vi "FPGAController_v4.2.vi"() -> ()   [LabVIEW 2015]
uses:
  <vilib>/Utility/miscctls.llb/LVPointTypeDef.ctl
  <vilib>/FPGAPlugInAG/PXIe-7971R/niLvFpga_Open_PXIe-7971R.vi
  <userlib>/_OpenG.lib/file/file.llb/Strip Path Extension - Path__ogtk.vi
  <userlib>/_OpenG.lib/comparison/comparison.llb/DBL Changed__ogtk.vi
  <userlib>/_OpenG.lib/comparison/comparison.llb/Boolean Changed__ogtk.vi
  <vilib>/Utility/error.llb/Error Cluster From Error Code.vi
  <vilib>/rvi/errors/niLvFpgaAdjustHostInterfaceError.vi
  <vilib>/addons/database/Connection.llb/Conn Execute.vi
  <vilib>/addons/database/Recordset.llb/Rec Fetch Recordset Data (R).vi
  <vilib>/addons/database/Recordset.llb/Rec Destroy - Connection.vi
  <vilib>/FPGAPlugInAG/PXIe-7971R/niLvFpga_Close_PXIe-7971R.vi
  <vilib>/rvi/interface/nirviOpenFPGA/nirviOpenFPGA.xnode
  FPGA Bitfiles/FPGAnew_FPGATarget_FPGAcode2_56iu3K9+1SM.lvbitx
  <vilib>/rvi/interface/nirviMethod/nirviMethod.xnode
  <vilib>/FPGA/interface/niFpgaViExecutionMode.ctl
  <vilib>/rvi/interface/nirviReadWriteControl/nirviReadWriteControl.xnode
  <vilib>/addons/database/_DB Variant To Data/Database Variant To Data.xnode
  <vilib>/rvi/interface/nirviCloseFPGA/nirviCloseFPGA.xnode
  <vilib>/addons/database/NI_Database_API.lvlib
  NiFpgaLv.dll
panel:
  in  "Tab Control":enum32{"Auto Threshold", "Manual Threshold"}(tab)
  in  "Refresh PSU":bool=TRUE
  in  "Auto Threshold":bool
  in  "Update All":bool
  in  "Raise Threshold":bool
  in  "Lower Threshold":bool
  in  "Threshold 1":bool
  in  "Threshold 2":bool
  in  "Threshold 3":bool
  in  "Threshold 4":bool
  in  "Threshold 5":bool
  in  "Threshold 6":bool
  in  "Threshold 7":bool
  in  "Update By":i32
  out "Time Betwee Shots":dbl
  out "Del Armed":bool
  out "Update Threshold":bool
  in  "Min. Time\nBetween Shots (s)":dbl
  in  "Rate Limiting":bool
  out "Armed":bool
  in  "Add Delay":bool
  in  "Delay Name":string
  in  "Delay Value":dbl=3.0 min=0.0
  in  "Delay Ring":dbl(ring)=3.15039 items=["Custom"]
  in  "Rearm Trigger":bool
  in  "One Shot Mode":bool
  out "Last Update:":timestamp
  out "Updating FPGA":bool
  out "Sensitivity":dbl
  out "error out":errorcluster
  out "Low Mass Limit":fxp<+,31,17>
  out "High Mass Limit":fxp<+,31,17>
  out "stopping":bool
  out "Peletron (MV)":dbl=2.0
  out "High Mass (kg)":dbl=inf
  out "Low Mass (kg)":dbl
  out "High Charge Limit":i16
  out "Low Charge Limit":i16
  out "High velocity count":i32=210
  out "Low velocity count":i32=21000
  in  "stop":bool
  in  "Peak-Threshold Factor":dbl=2.0
  out "Low Charge Limit (fC)":dbl
  out "High Charge Limit (fC)":dbl=100.0
  out "High Velocity":dbl=100000.0
  out "Low Velocity":dbl=1000.0
  out "Filter 7 Peak":i32=7483
  out "Filter 6 Peak":i32=9863
  out "Filter 5 Peak":i32=13910
  out "Filter 4 Peak":i32=18191
  out "Filter 3 Peak":i32=46254
  out "Filter 2 Peak":i32=120664
  out "Filter 1 Peak":i32=295996
  in  "Filter7 Threshold":i32=-21165
  in  "Filter6 Threshold":i32=-29358
  in  "Filter5 Threshold":i32=-41730
  in  "Filter4 Threshold":i32=-54306
  in  "Filter3 Threshold":i32=-138762
  in  "Filter2 Threshold":i32=-361992
  in  "Filter1 Threshold":i32=-887988
  in  "Zero Peak Values":bool
  in  "Assign Threshold":bool
  in  "Run Mode":bool
  # "Settings"
  # "Dubugging"
  # "Independent Variable"
  # "Low Vel."
  # "High Vel."
  # "Low Q (fC)"
  # "High Q (fC)"
  # "Plate Control While Loop Counter"
  # "Low Mass (kg)"
  # "High Mass (kg)"
  # "Sens. (V/pC)"
  # "Peletron (MV)"
  # "Current Value of Running Average"
  # "Peak Threshold Factor"
  # "Delay Trigger"
  # "Dist. from 2nd Det. (m)"
  # "Name"
  # "Peak Values"
  # "Peak 1"
  # "Peak 2"
  # "Peak 3"
  # "Peak 4"
  # "Peak 5"
  # "Peak 6"
  # "Peak 7"
  # "Thresholds"
  # "Threshold 1"
  # "Threshold 2"
  # "Threshold 3"
  # "Threshold 4"
  # "Threshold 5"
  # "Threshold 6"
  # "Threshold 7"
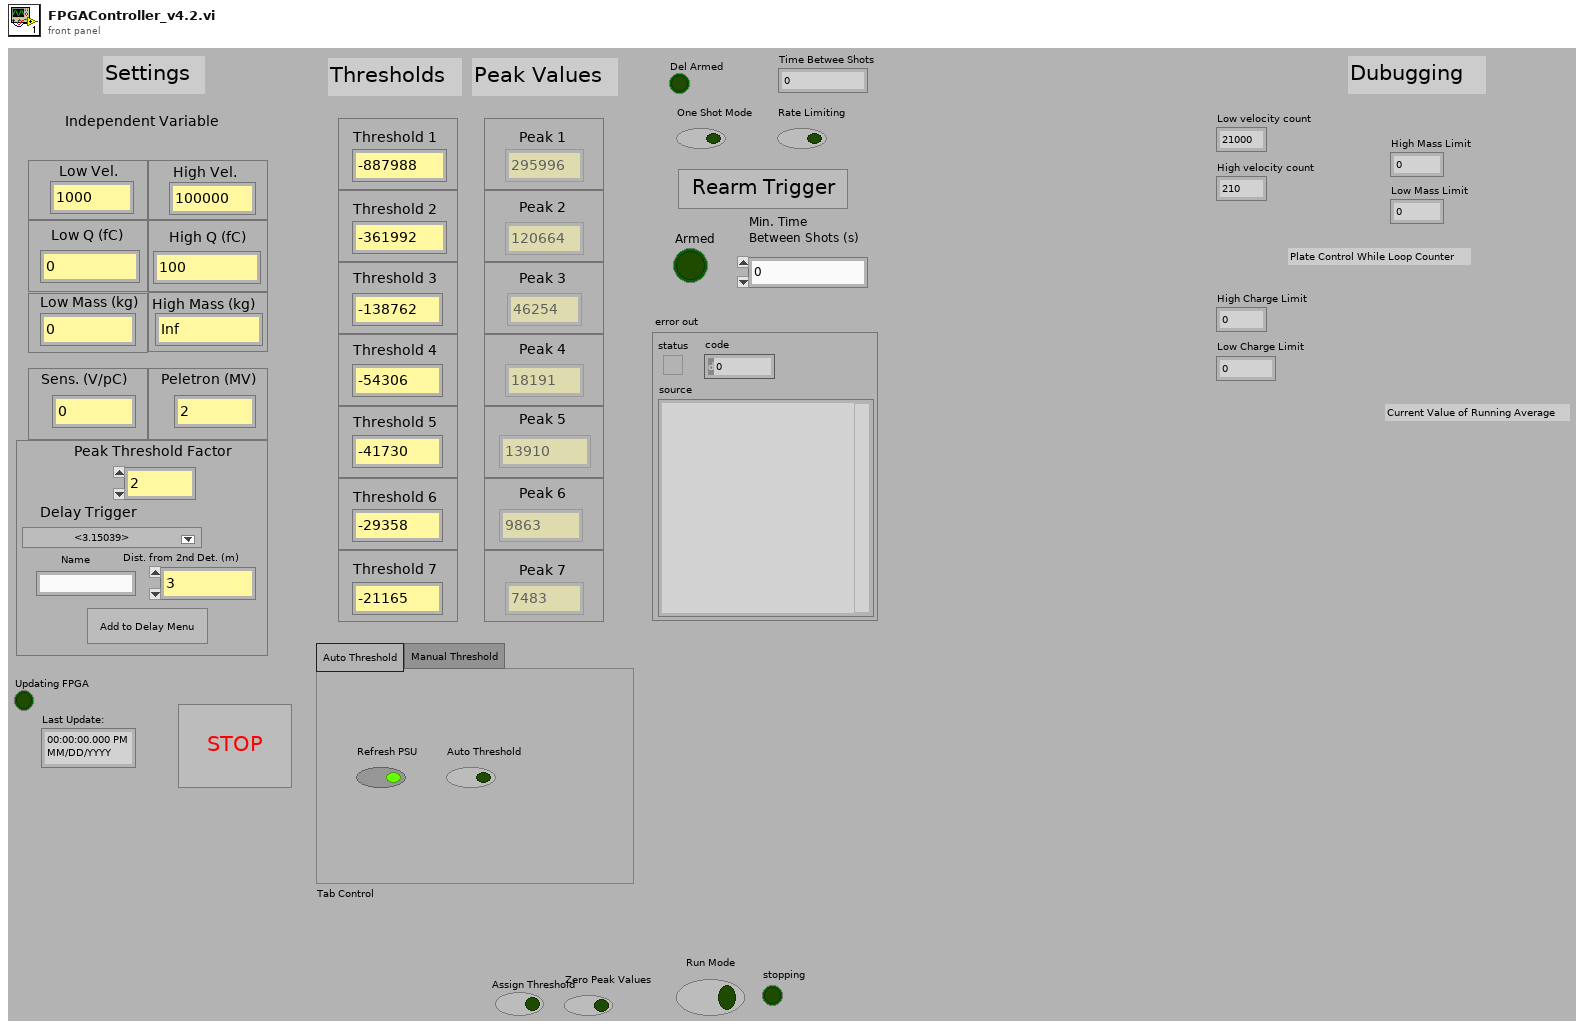
[diagram p1: front panel]
types:
  T1 = typedef "LVPointTypeDef.ctl" = cluster{"Horizontal":i16, "Vertical":i16}
  T2 = enum8{"Enabled", "Disabled", "Disabled and Grayed Out"}
  T3 = typedef "NI_Database_API.lvlib/Conn ObjectReference.ctl" = refnum<k1>
  T4 = typedef "NI_Database_API.lvlib/Rec ObjectReference.ctl" = refnum<k1>
  T5 = cluster{"Filter 1 Peak":i32, "Filter 2 Peak":i32, "Filter 3 Peak":i32, "Filter 4 Peak":i32, "Filter 5 Peak":i32, "Filter 6 Peak":i32, "Filter 7 Peak":i32}
  T6 = typedef "LVStringsAndValuesArrayTypeDef_DBL.ctl" = cluster{"String":string, "Value":dbl}[]
  T7 = cluster{"Numeric":dbl, "Numeric":dbl, "Numeric":dbl, "Numeric":dbl, "Numeric":dbl, "Numeric":dbl, i32, dbl, "Value":dbl, fxp<+,16,7>, bool}
  T8 = cluster{"Low Velocity Count":i32, "High Velocity Count":i32, "Low Charge Limit (ADC ticks)":i16, "High Charge Limit (ADC ticks)":i16, "Low Mass (ADC*cycle^2)":i64, "High Mass (ADC*cycle^2)":i64, "Mult":fxp<+,16,7>, "Mult Use?":bool}
  T9 = cluster{"Filter 1 Detector 3 Correlation":i32, "Filter 2 Detector 3 Correlation":i32, "Filter 3 Detector 3 Correlation":i32, "Filter 4 Detector 3 Correlation":i32, "Filter 5 Detector 3 Correlation":i32, "Filter 6 Detector 3 Correlation":i32, "Filter 7 Detector 3 Correlation":i32}
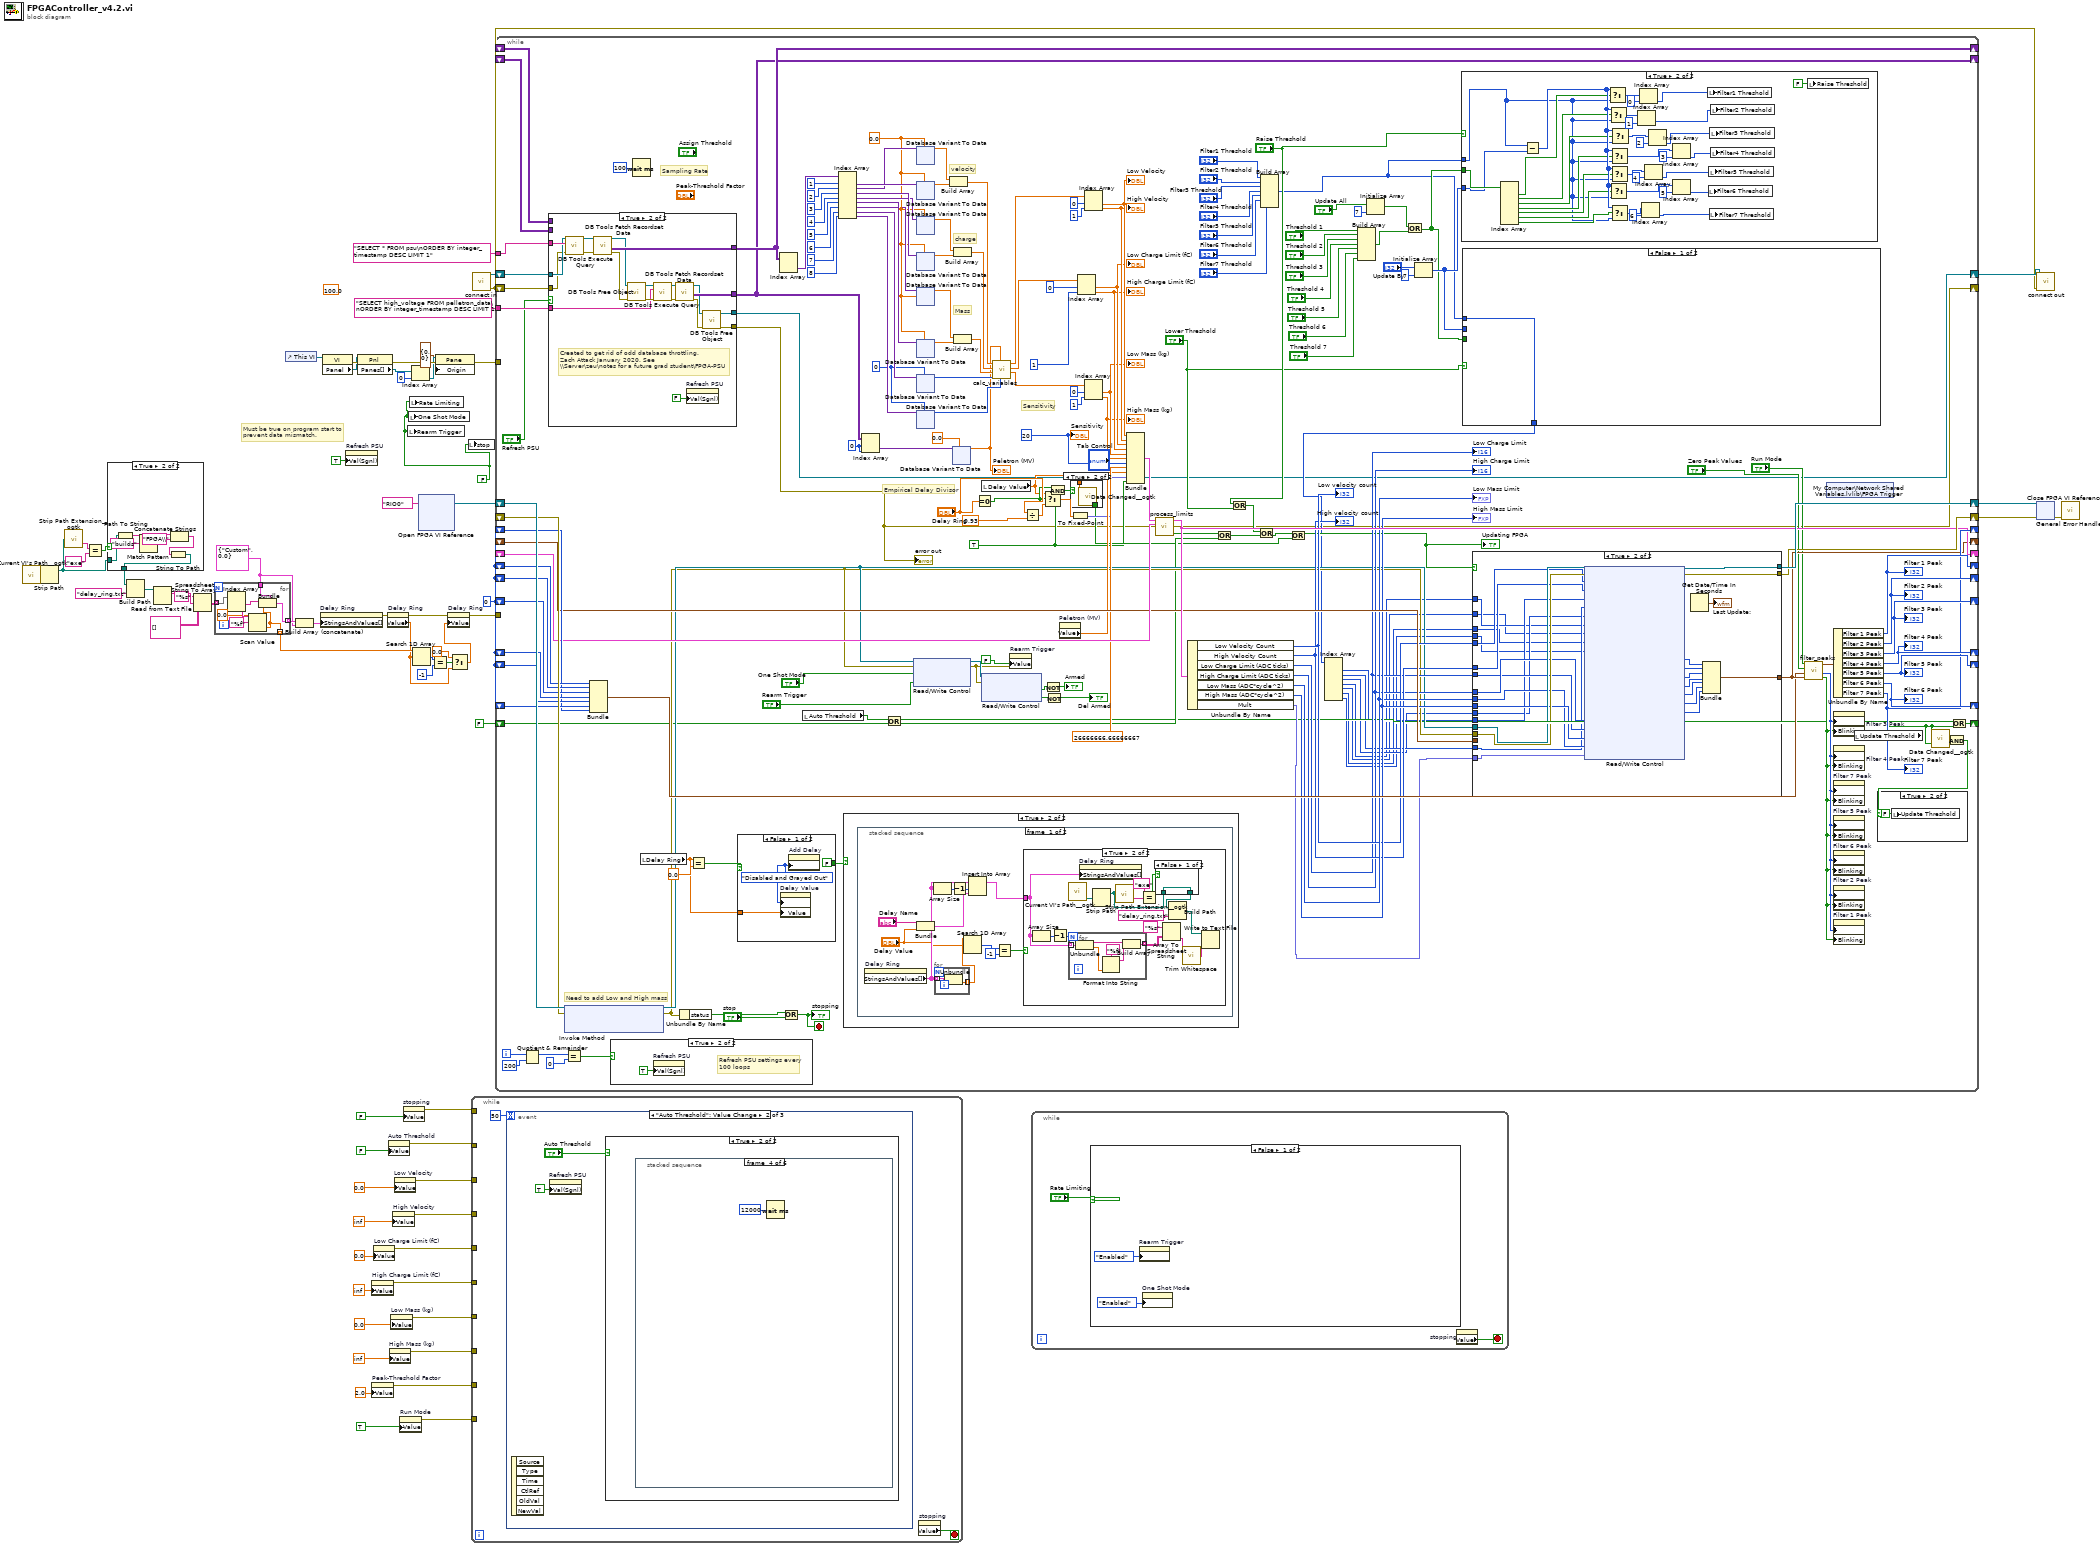
[diagram p0: block diagram]
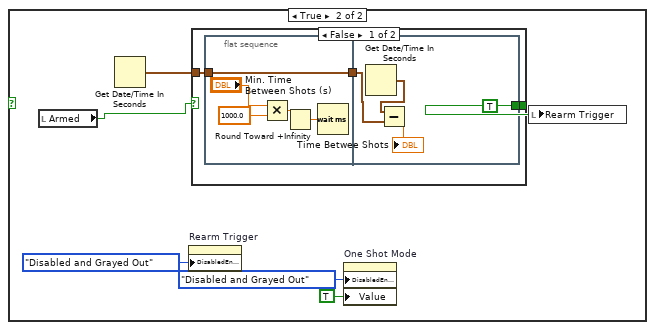
[diagram p3: hidden frame]
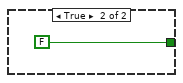
[diagram p4: hidden frame]
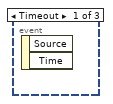
[diagram p5: hidden frame]
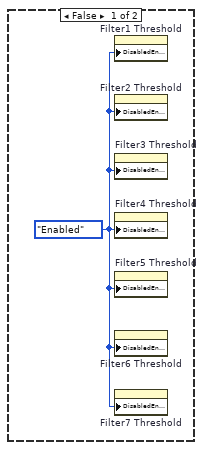
[diagram p6: hidden frame]
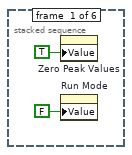
[diagram p7: hidden frame]
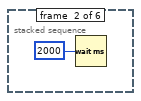
[diagram p8: hidden frame]
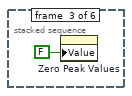
[diagram p9: hidden frame]
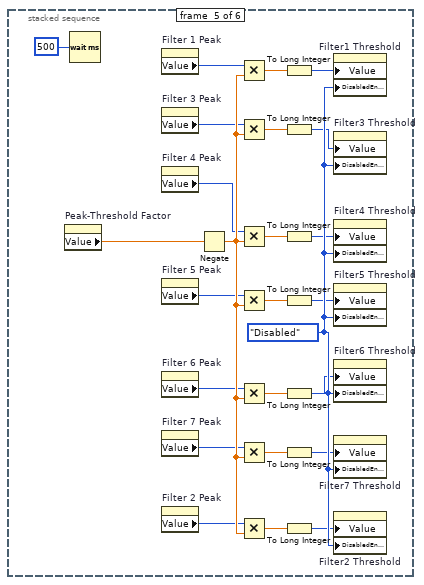
[diagram p10: hidden frame]
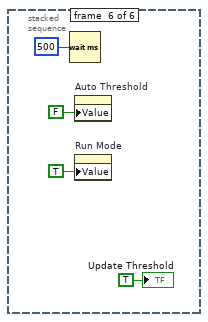
[diagram p11: hidden frame]
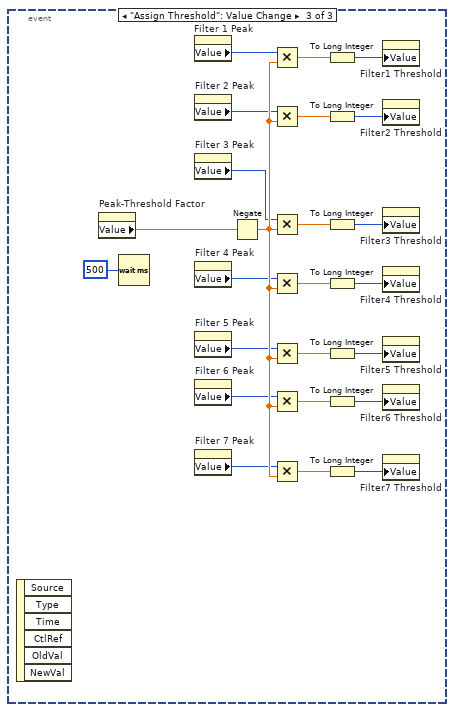
[diagram p12: hidden frame]
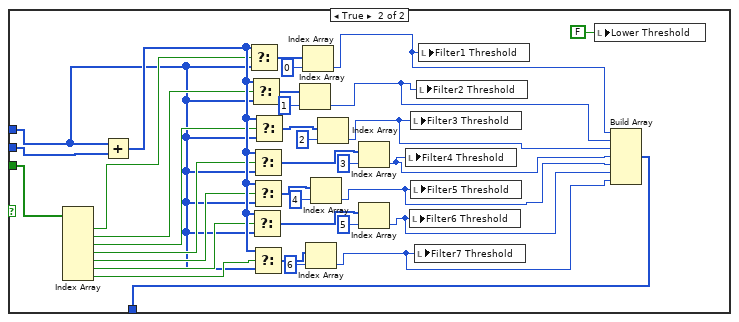
[diagram p15: hidden frame]
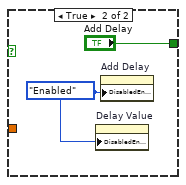
[diagram p19: hidden frame]
diagram:
  (unwired) 100.0 ("Update By")
  w19 = cluster{"String":string, "Value":dbl} {"String"="Custom", "Value"=0.0}
  w29 = FALSE
  w67 = 0
  # "Must be true on program start to\nprevent data mismatch."
  n1 = call <userlib>:"Current VI's Path__ogtk.vi"() -> ("Current VI's Path (+ Relative)"=w28:path)  [unwired: 1 in]
  n2 = Strip Path(path=w28) -> (stripped path=w14:path)  [unwired: 1 out]
  n3 = call-poly <userlib>:"Strip Path Extension__ogtk.vi"("path"=w14) -> ("extension"=w18:string)  [unwired: 1 out]
  n4 = Equal?(x=w18, y="exe") -> (x = y?=w15:bool)
  n5 = case shown="True" w15 {
    tunnel: w14 -> [w69 w76]
    tunnel: [w69 w70] -> w13
    frame False {
    }
    frame True {
      n6 = Path To String(path=w76) -> (string=w75:string)
      n7 = Match Pattern(string=w75, regular expression="builds") -> (before substring=w73:string)  [unwired: 1 in, 3 out]
      n8 = Concatenate Strings(w73, "FPGA\\" ("string")) -> (w71:string)
      n9 = String To Path(string=w71) -> (path=w70:path)
    }
  }
  n10 = Build Path(base path=w13, name or relative path="delay_ring.txt") -> (appended path=w16:path)
  n11 = Read from Text File(file (use dialog)=w16) -> (text=w26:string)  [unwired: 3 in, 3 out]
  n12 = Spreadsheet String To Array(format string="%s", spreadsheet string=w26, array type (2D Dbl)=string[][] []) -> (array=w23:string[][])  [unwired: 1 in]
  n13 = for {
    tunnel: w23 -> [w84] mode=indexing
    tunnel: w19 -> [w82]
    tunnel: [w78] -> w20 mode=indexing
    tunnel: [w77] -> w12 mode=indexing
    n14 = Index Array(array=w84) -> (element #1=w83:string, element #2=w81:string)  [unwired: 2 in]
    n15 = Scan Value(string=w81, format string="%f", default (0 dbl)=0.0) -> (value=w77:dbl)  [unwired: 1 out]
    n16 = Bundle(cluster=w82, "String"=w83, "Value"=w77) -> (w78:cluster{"String":string, "Value":dbl})
  }
  n17 = control-ref of="This VI"() -> (w40:refnum<vi>)
  n18 = Build Array (concatenate)(w20, w19) -> (w22:cluster{"String":string, "Value":dbl}[])
  n19 = property on="Delay Ring" class="Ring (strict)"("StringsAndValues[]"=w22) -> (error out=w21:errorcluster)  [unwired: 2 in, 1 out]
  n20 = property class="VI"(reference=w40) -> (error out=w39:errorcluster, "Panel"=w38:refnum<vi>)  [unwired: 1 in, 1 out]
  n21 = property on="Refresh PSU" class="Bool (strict)"("Val(Sgnl)"=TRUE ("Value (Signaling)")) -> ()  [unwired: 2 in, 2 out]
  n22 = property class="Pnl"(reference=w38, error in=w39) -> (error out=w37:errorcluster, "Panes[]"=w36:refnum<vi>[])  [unwired: 1 out]
  n23 = property on="High Charge Limit (fC)" class="DigNum (strict)"("Value"=inf ("High Charge Limit (fC)")) -> (error out=w54:errorcluster)  [unwired: 2 in, 1 out]
  n24 = property on="Peak-Threshold Factor" class="DigNum (strict)"("Value"=2.0 ("Peak-Threshold Factor")) -> (error out=w48:errorcluster)  [unwired: 2 in, 1 out]
  n25 = property on="Low Charge Limit (fC)" class="DigNum (strict)"("Value"=0.0 ("Low Charge Limit (fC)")) -> (error out=w56:errorcluster)  [unwired: 2 in, 1 out]
  n26 = property on="Delay Ring" class="Ring (strict)"(error in=w21) -> (error out=w11:errorcluster, "Value"=w5:dbl)  [unwired: 1 in, 1 out]
  n27 = property on="Auto Threshold" class="Bool (strict)"("Value"=FALSE ("Auto Threshold")) -> (error out=w62:errorcluster)  [unwired: 2 in, 1 out]
  n28 = property on="High Mass (kg)" class="DigNum (strict)"("Value"=inf ("High Mass (kg)")) -> (error out=w50:errorcluster)  [unwired: 2 in, 1 out]
  n29 = property on="Low Mass (kg)" class="DigNum (strict)"("Value"=0.0 ("Low Mass (kg)")) -> (error out=w52:errorcluster)  [unwired: 2 in, 1 out]
  n30 = property on="High Velocity" class="DigNum (strict)"("Value"=inf ("High Velocity")) -> (error out=w58:errorcluster)  [unwired: 2 in, 1 out]
  n31 = property on="Low Velocity" class="DigNum (strict)"("Value"=0.0 ("Low Velocity")) -> (error out=w60:errorcluster)  [unwired: 2 in, 1 out]
  n32 = property on="Run Mode" class="Bool (strict)"("Value"=TRUE ("Run Mode")) -> (error out=w46:errorcluster)  [unwired: 2 in, 1 out]
  n33 = property on="stopping" class="Bool (strict)"("Value"=FALSE ("stopping")) -> (error out=w64:errorcluster)  [unwired: 2 in, 1 out]
  n34 = local write "Rearm Trigger"(w29) -> ()
  n35 = local write "One Shot Mode"(w29) -> ()
  n36 = local write "Rate Limiting"(w29) -> ()
  n37 = Index Array(array=w36, index=0) -> (element=w34:refnum<vi>)
  n38 = Search 1D Array(1D array=w12, element=w5) -> (index of element=w9:i32)  [unwired: 1 in]
  n39 = xnode "Open FPGA VI Reference"("resource name"=tag "RIO0") -> ("FPGA VI Reference Out"=w31:refnum<k20>)  [unwired: 1 in, 1 out]
  n40 = Equal?(x=w9, y=-1) -> (x = y?=w7:bool)
  n41 = property class="Pane"(reference=w34, error in=w37, "Origin"=T1 {"Horizontal"=0, "Vertical"=0}) -> (error out=w32:errorcluster)  [unwired: 1 out]
  n42 = Select(t=0.0, s=w7, f=w5) -> (s? t:f=w6:dbl)
  n43 = property on="Delay Ring" class="Ring (strict)"(error in=w11, "Value"=w6) -> (error out=w10:errorcluster)  [unwired: 1 in, 1 out]
  n44 = local write "stop"(w29) -> ()
  n45 = while {
    tunnel: w64 -> [_]
    tunnel: w62 -> [_]
    tunnel: w60 -> [_]
    tunnel: w58 -> [_]
    tunnel: w56 -> [_]
    tunnel: w54 -> [_]
    tunnel: w52 -> [_]
    tunnel: w50 -> [_]
    tunnel: w48 -> [_]
    tunnel: w46 -> [_]
    stop <- w86 stop-if-true
    n46 = event shown="[1] \"Auto Threshold\": Value Change" {
      selector: _ -> [_ _ _]
      dyn-events: _ -> [_ _ _]
      timeout: 50 -> [_ _ _]
      event Timeout {
        n47 = event-data() -> ()  [unwired: 1 in, 2 out]
      }
      event "Auto Threshold": Value Change {
        n48 = event-data() -> ()  [unwired: 1 in, 6 out]
        n49 = property on="Refresh PSU" class="Bool (strict)"("Val(Sgnl)"=TRUE ("Value (Signaling)")) -> ()  [unwired: 2 in, 2 out]
        n50 = case shown="True" "Auto Threshold" {
          frame False {
            w89 = T2."Enabled" ("Disabled")
            n51 = property on="Filter1 Threshold" class="DigNum (strict)"("DisabledEnum"=w89) -> ()  [unwired: 2 in, 2 out]
            n52 = property on="Filter2 Threshold" class="DigNum (strict)"("DisabledEnum"=w89) -> ()  [unwired: 2 in, 2 out]
            n53 = property on="Filter3 Threshold" class="DigNum (strict)"("DisabledEnum"=w89) -> ()  [unwired: 2 in, 2 out]
            n54 = property on="Filter4 Threshold" class="DigNum (strict)"("DisabledEnum"=w89) -> ()  [unwired: 2 in, 2 out]
            n55 = property on="Filter5 Threshold" class="DigNum (strict)"("DisabledEnum"=w89) -> ()  [unwired: 2 in, 2 out]
            n56 = property on="Filter6 Threshold" class="DigNum (strict)"("DisabledEnum"=w89) -> ()  [unwired: 2 in, 2 out]
            n57 = property on="Filter7 Threshold" class="DigNum (strict)"("DisabledEnum"=w89) -> ()  [unwired: 2 in, 2 out]
          }
          frame True {
            n58 = stacked-sequence {
              frame #0 {
                n59 = property on="Zero Peak Values" class="Bool (strict)"("Value"=TRUE ("Zero Peak Values")) -> ()  [unwired: 2 in, 2 out]
                n60 = property on="Run Mode" class="Bool (strict)"("Value"=FALSE ("Run Mode")) -> ()  [unwired: 2 in, 2 out]
              }
              frame #1 {
                n61 = Wait (ms)(milliseconds to wait=u32 2000) -> ()  [unwired: 1 out]
              }
              frame #2 {
                n62 = property on="Zero Peak Values" class="Bool (strict)"("Value"=FALSE ("Zero Peak Values")) -> ()  [unwired: 2 in, 2 out]
              }
              frame #3 {
                n63 = Wait (ms)(milliseconds to wait=u32 12000) -> ()  [unwired: 1 out]
              }
              frame #4 {
                w119 = T2."Disabled" ("Disabled")
                n64 = property on="Peak-Threshold Factor" class="DigNum (strict)"() -> ("Value"=w104:dbl)  [unwired: 2 in, 2 out]
                n65 = Wait (ms)(milliseconds to wait=u32 500) -> ()  [unwired: 1 out]
                n66 = property on="Filter 1 Peak" class="DigNum (strict)"() -> ("Value"=w102:i32)  [unwired: 2 in, 2 out]
                n67 = property on="Filter 3 Peak" class="DigNum (strict)"() -> ("Value"=w100:i32)  [unwired: 2 in, 2 out]
                n68 = property on="Filter 4 Peak" class="DigNum (strict)"() -> ("Value"=w99:i32)  [unwired: 2 in, 2 out]
                n69 = property on="Filter 5 Peak" class="DigNum (strict)"() -> ("Value"=w98:i32)  [unwired: 2 in, 2 out]
                n70 = property on="Filter 6 Peak" class="DigNum (strict)"() -> ("Value"=w97:i32)  [unwired: 2 in, 2 out]
                n71 = property on="Filter 7 Peak" class="DigNum (strict)"() -> ("Value"=w96:i32)  [unwired: 2 in, 2 out]
                n72 = property on="Filter 2 Peak" class="DigNum (strict)"() -> ("Value"=w101:i32)  [unwired: 2 in, 2 out]
                n73 = Negate(x=w104) -> (-x=w103:dbl)
                n74 = Multiply(x=w102, y=w103) -> (x*y=w118:dbl)
                n75 = Multiply(x=w100, y=w103) -> (x*y=w114:dbl)
                n76 = Multiply(x=w99, y=w103) -> (x*y=w112:dbl)
                n77 = Multiply(x=w98, y=w103) -> (x*y=w110:dbl)
                n78 = Multiply(x=w97, y=w103) -> (x*y=w108:dbl)
                n79 = Multiply(x=w96, y=w103) -> (x*y=w106:dbl)
                n80 = Multiply(x=w101, y=w103) -> (x*y=w116:dbl)
                n81 = To Long Integer(number=w118) -> (32bit integer=w117:i32)
                n82 = To Long Integer(number=w114) -> (32bit integer=w113:i32)
                n83 = To Long Integer(number=w112) -> (32bit integer=w111:i32)
                n84 = To Long Integer(number=w110) -> (32bit integer=w109:i32)
                n85 = To Long Integer(number=w108) -> (32bit integer=w107:i32)
                n86 = To Long Integer(number=w106) -> (32bit integer=w105:i32)
                n87 = To Long Integer(number=w116) -> (32bit integer=w115:i32)
                n88 = property on="Filter1 Threshold" class="DigNum (strict)"("Value"=w117, "DisabledEnum"=w119) -> ()  [unwired: 2 in, 2 out]
                n89 = property on="Filter3 Threshold" class="DigNum (strict)"("Value"=w113, "DisabledEnum"=w119) -> ()  [unwired: 2 in, 2 out]
                n90 = property on="Filter4 Threshold" class="DigNum (strict)"("Value"=w111, "DisabledEnum"=w119) -> ()  [unwired: 2 in, 2 out]
                n91 = property on="Filter5 Threshold" class="DigNum (strict)"("Value"=w109, "DisabledEnum"=w119) -> ()  [unwired: 2 in, 2 out]
                n92 = property on="Filter6 Threshold" class="DigNum (strict)"("Value"=w107, "DisabledEnum"=w119) -> ()  [unwired: 2 in, 2 out]
                n93 = property on="Filter7 Threshold" class="DigNum (strict)"("Value"=w105, "DisabledEnum"=w119) -> ()  [unwired: 2 in, 2 out]
                n94 = property on="Filter2 Threshold" class="DigNum (strict)"("Value"=w115, "DisabledEnum"=w119) -> ()  [unwired: 2 in, 2 out]
              }
              frame #5 {
                n95 = Wait (ms)(milliseconds to wait=u32 500) -> ()  [unwired: 1 out]
                n96 = property on="Auto Threshold" class="Bool (strict)"("Value"=FALSE ("Auto Threshold")) -> ()  [unwired: 2 in, 2 out]
                n97 = property on="Run Mode" class="Bool (strict)"("Value"=TRUE ("Run Mode")) -> ()  [unwired: 2 in, 2 out]
                "Update Threshold" <- TRUE ("Update Threshold")
              }
            }
          }
        }
      }
      event "Assign Threshold": Value Change {
        n98 = event-data() -> ()  [unwired: 1 in, 6 out]
        n99 = property on="Peak-Threshold Factor" class="DigNum (strict)"() -> ("Value"=w138:dbl)  [unwired: 2 in, 2 out]
        n100 = Wait (ms)(milliseconds to wait=u32 500) -> ()  [unwired: 1 out]
        n101 = property on="Filter 1 Peak" class="DigNum (strict)"() -> ("Value"=w137:i32)  [unwired: 2 in, 2 out]
        n102 = property on="Filter 2 Peak" class="DigNum (strict)"() -> ("Value"=w136:i32)  [unwired: 2 in, 2 out]
        n103 = property on="Filter 3 Peak" class="DigNum (strict)"() -> ("Value"=w135:i32)  [unwired: 2 in, 2 out]
        n104 = property on="Filter 4 Peak" class="DigNum (strict)"() -> ("Value"=w134:i32)  [unwired: 2 in, 2 out]
        n105 = property on="Filter 5 Peak" class="DigNum (strict)"() -> ("Value"=w133:i32)  [unwired: 2 in, 2 out]
        n106 = property on="Filter 6 Peak" class="DigNum (strict)"() -> ("Value"=w132:i32)  [unwired: 2 in, 2 out]
        n107 = property on="Filter 7 Peak" class="DigNum (strict)"() -> ("Value"=w131:i32)  [unwired: 2 in, 2 out]
        n108 = Negate(x=w138) -> (-x=w140:dbl)
        n109 = Multiply(x=w137, y=w140) -> (x*y=w147:dbl)
        n110 = Multiply(x=w136, y=w140) -> (x*y=w145:dbl)
        n111 = Multiply(x=w135, y=w140) -> (x*y=w144:dbl)
        n112 = Multiply(x=w134, y=w140) -> (x*y=w143:dbl)
        n113 = Multiply(x=w133, y=w140) -> (x*y=w142:dbl)
        n114 = Multiply(x=w132, y=w140) -> (x*y=w141:dbl)
        n115 = Multiply(x=w131, y=w140) -> (x*y=w146:dbl)
        n116 = To Long Integer(number=w147) -> (32bit integer=w130:i32)
        n117 = To Long Integer(number=w145) -> (32bit integer=w129:i32)
        n118 = To Long Integer(number=w144) -> (32bit integer=w128:i32)
        n119 = To Long Integer(number=w143) -> (32bit integer=w127:i32)
        n120 = To Long Integer(number=w142) -> (32bit integer=w126:i32)
        n121 = To Long Integer(number=w141) -> (32bit integer=w125:i32)
        n122 = To Long Integer(number=w146) -> (32bit integer=w124:i32)
        n123 = property on="Filter1 Threshold" class="DigNum (strict)"("Value"=w130) -> ()  [unwired: 2 in, 2 out]
        n124 = property on="Filter2 Threshold" class="DigNum (strict)"("Value"=w129) -> ()  [unwired: 2 in, 2 out]
        n125 = property on="Filter3 Threshold" class="DigNum (strict)"("Value"=w128) -> ()  [unwired: 2 in, 2 out]
        n126 = property on="Filter4 Threshold" class="DigNum (strict)"("Value"=w127) -> ()  [unwired: 2 in, 2 out]
        n127 = property on="Filter5 Threshold" class="DigNum (strict)"("Value"=w126) -> ()  [unwired: 2 in, 2 out]
        n128 = property on="Filter6 Threshold" class="DigNum (strict)"("Value"=w125) -> ()  [unwired: 2 in, 2 out]
        n129 = property on="Filter7 Threshold" class="DigNum (strict)"("Value"=w124) -> ()  [unwired: 2 in, 2 out]
      }
    }
    n130 = property on="stopping" class="Bool (strict)"() -> ("Value"=w86:bool)  [unwired: 2 in, 2 out]
  }
  n131 = call "connect in.vi"() -> ("error out"=w41:errorcluster, "Database Connection"=w42:T3)  [unwired: 7 in, 1 out]
  n132 = while {
    shift-right: [w321] -> w66
    shift-left: w31 -> [w325]
    shift-right: [w320] -> w65
    shift-left: _ -> [w324]
    shift-right: [w316] -> _
    shift-left: w67 -> [w309]
    shift-right: [w315] -> _
    shift-left: w67 -> [w308]
    shift-right: [w314] -> _
    shift-left: w67 -> [w307]
    shift-right: [w313] -> _
    shift-left: w67 -> [w306]
    shift-right: [w312] -> _
    shift-left: w67 -> [w305]
    shift-right: [w318] -> _
    shift-left: w67 -> [w311]
    shift-right: [w317] -> _
    shift-left: w67 -> [w310]
    tunnel: "SELECT * FROM psu\nORDER BY integer_timestamp DESC LIMIT 1" ("SQL query") -> [w163]
    shift-right: [w159] -> w43
    shift-left: w42 -> [w162]
    shift-right: [w158] -> _
    shift-left: w41 -> [w161]
    shift-right: [w304] -> _
    shift-left: _ -> [w303]
    shift-right: [w301] -> _
    shift-left: _ -> [w302]
    tunnel: w32 -> [_]
    tunnel: w10 -> [_]
    shift-right: [w217] -> _
    shift-left: FALSE -> [w220]
    tunnel: "SELECT high_voltage FROM pelletron_data\nORDER BY integer_timestamp DESC LIMIT 1" ("SQL query") -> [w160]
    shift-right: [w157] -> _
    shift-left: _ -> [w156]
    shift-right: [w155] -> _
    shift-left: _ -> [w154]
    i -> [w152]
    stop <- w319 stop-if-true
    w185 = TRUE
    w267 = 0 ("index (row)")
    w268 = i8 0
    w269 = 0.0
    w243 = 20
    # "charge"
    # "Empirical Delay Divisor"
    # "Mass"
    # "velocity"
    # "Sensitivity"
    # "Sampling Rate"
    # "Need to add Low and High mass"
    n133 = Quotient & Remainder(x=w152, y=200) -> (x-y*floor(x/y)=w150:i32)  [unwired: 1 out]
    n134 = case shown="True" "Refresh PSU" {
      tunnel: [w328 w347] -> w157
      tunnel: w163 -> [_ w346]
      tunnel: w162 -> [w330 w345]
      tunnel: w161 -> [w329 w344]
      tunnel: w160 -> [_ w337]
      tunnel: [w327 w336] -> w155
      tunnel: [w330 w333] -> w159
      tunnel: [w329 w332] -> w158
      tunnel: w156 -> [w328 _]
      tunnel: w154 -> [w327 _]
      frame False {
      }
      frame True {
        # "Created to get rid of odd database throttling.\nZach Attack January 2020. See \n\\\\Server\\zeu\\notes for a future grad student\\FPGA-PSU"
        n135 = call-poly <vilib>:"DB Tools Execute Query.vi"("error in (no error)"=w344, "SQL query"=w346, "connection reference"=w345) -> ("error out"=w348:errorcluster, "recordset reference"=w349:T4)  [unwired: 5 in]
        n136 = call-poly <vilib>:"DB Tools Fetch Recordset Data.vi"("error in (no error)"=w348, "recordset reference"=w349) -> ("error out"=w338:errorcluster, "recordset data"=w347:variant[][], "recordset reference out"=w341:T4)  [unwired: 3 in]
        n137 = call-poly <vilib>:"DB Tools Free Object.vi"("error in (no error)"=w338, "recordset reference"=w341) -> ("error out"=w339:errorcluster, "connection reference"=w340:T3)  [unwired: 8 in]
        n138 = call-poly <vilib>:"DB Tools Execute Query.vi"("error in (no error)"=w339, "SQL query"=w337, "connection reference"=w340) -> ("error out"=w343:errorcluster, "recordset reference"=w342:T4)  [unwired: 5 in]
        n139 = call-poly <vilib>:"DB Tools Fetch Recordset Data.vi"("error in (no error)"=w343, "recordset reference"=w342) -> ("error out"=w334:errorcluster, "recordset data"=w336:variant[][], "recordset reference out"=w335:T4)  [unwired: 3 in]
        n140 = property on="Refresh PSU" class="Bool (strict)"("Val(Sgnl)"=FALSE ("Value (Signaling)")) -> ()  [unwired: 2 in, 2 out]
        n141 = call-poly <vilib>:"DB Tools Free Object.vi"("error in (no error)"=w334, "recordset reference"=w335) -> ("error out"=w332:errorcluster, "connection reference"=w333:T3)  [unwired: 8 in]
      }
    }
    "error out" <- w158
    n142 = xnode "Invoke Method"("FPGA VI Reference In"=w325, "error in"=w324) -> ("FPGA VI Reference Out"=w237:refnum<k20>, "error out"=w236:errorcluster)  [unwired: 1 out]
    n143 = Equal?(x=w150, y=0) -> (x = y?=w148:bool)
    n144 = Bundle("Filter 1 Peak"=w311, "Filter 2 Peak"=w310, "Filter 3 Peak"=w309, "Filter 4 Peak"=w308, "Filter 5 Peak"=w307, "Filter 6 Peak"=w306, "Filter 7 Peak"=w305) -> (w297:T5)  [unwired: 1 in]
    n145 = case shown="True" w148 {
      frame False {
      }
      frame True {
        # "Refresh PSU settings every\n100 loops"
        n146 = property on="Refresh PSU" class="Bool (strict)"("Val(Sgnl)"=TRUE ("Value (Signaling)")) -> ()  [unwired: 2 in, 2 out]
      }
    }
    n147 = Wait (ms)(milliseconds to wait=u32 100) -> ()  [unwired: 1 out]
    n148 = local read "Delay Ring"() -> (w221:dbl)
    n149 = Unbundle By Name(w236) -> ("status"=w323:bool)
    n150 = Equal?(x=w221, y=0.0) -> (x = y?=w222:bool)
    n151 = case shown="False" w222 {
      tunnel: [FALSE ("Add Delay") "Add Delay"] -> w240
      tunnel: w221 -> [w423 _]
      frame False {
        w424 = T2."Disabled and Grayed Out" ("Disabled")
        n152 = property on="Delay Value" class="DigNum (strict)"("DisabledEnum"=w424, "Value"=w423) -> ()  [unwired: 2 in, 2 out]
        n153 = property on="Add Delay" class="Bool (strict)"("DisabledEnum"=w424) -> ()  [unwired: 2 in, 2 out]
      }
      frame True {
        w425 = T2."Enabled" ("Disabled")
        n154 = property on="Delay Value" class="DigNum (strict)"("DisabledEnum"=w425) -> ()  [unwired: 2 in, 2 out]
        n155 = property on="Add Delay" class="Bool (strict)"("DisabledEnum"=w425) -> ()  [unwired: 2 in, 2 out]
      }
    }
    n156 = Index Array(array=w157) -> (element=w278:variant[])  [unwired: 2 in]
    n157 = Or(x=w323, y="stop") -> (x .or. y?=w319:bool)
    "stopping" <- w319
    n158 = local read "Auto Threshold"() -> (w218:bool)
    n159 = Index Array(array=w278, index #1=1 ("index"), index #2=2 ("index"), index #3=3 ("index"), index #4=4 ("index"), index #5=5 ("index"), index #6=6 ("index"), index #7=7 ("index"), index #8=8 ("index")) -> (element #1=w277:variant, element #2=w276:variant, element #3=w275:variant, element #4=w274:variant, element #5=w273:variant, element #6=w272:variant, element #7=w271:variant, element #8=w270:variant)
    n160 = case shown="True" w240 {
      frame False {
      }
      frame True {
        n161 = stacked-sequence {
          frame #0 {
            n162 = property on="Delay Ring" class="Ring (strict)"() -> ("StringsAndValues[]"=w429:T6)  [unwired: 2 in, 2 out]
            n163 = Bundle("Delay Name"="Delay Name", "Delay Value"="Delay Value") -> (w434:cluster{"Delay Name":string, "Delay Value":dbl})  [unwired: 1 in]
            n164 = Array Size(array=w429) -> (size(s)=w432:i32)
            n165 = for {
              tunnel: w429 -> [w439] mode=indexing
              tunnel: [w438] -> w428 mode=indexing
              n166 = Unbundle(w439) -> ("Value"=w438:dbl)  [unwired: 1 out]
            }
            n167 = Decrement(x=w432) -> (x-1=w431:i32)
            n168 = Search 1D Array(1D array=w428, element="Delay Value") -> (index of element=w436:i32)  [unwired: 1 in]
            n169 = Insert Into Array(array=w429, index=w431, new element=w434) -> (w433:T6)
            n170 = Equal?(x=w436, y=-1) -> (x = y?=w430:bool)
            n171 = case shown="True" w430 {
              tunnel: w433 -> [_ w448]
              frame False {
                n172 = One Button Dialog(message="Value Already Exists") -> ()  [unwired: 1 in, 1 out]
              }
              frame True {
                n173 = Array Size(array=w448) -> (size(s)=w450:i32)
                n174 = Decrement(x=w450) -> (x-1=w449:i32)
                n175 = call <userlib>:"Current VI's Path__ogtk.vi"() -> ("Current VI's Path (+ Relative)"=w454:path)  [unwired: 1 in]
                n176 = for {
                  N: w449 -> [_]
                  tunnel: w448 -> [w464] mode=indexing
                  tunnel: [w459] -> w451 mode=indexing
                  n177 = Unbundle(w464) -> ("String"=w460:string, "Value"=w463:dbl)
                  n178 = Format Into String(format string="%f", w463) -> (resulting string=w461:string)  [unwired: 2 in, 1 out]
                  n179 = Build Array(w460, w461) -> (w459:string[])
                }
                n180 = property on="Delay Ring" class="Ring (strict)"("StringsAndValues[]"=w448) -> ()  [unwired: 2 in, 2 out]
                n181 = Strip Path(path=w454) -> (stripped path=w442:path)  [unwired: 1 out]
                n182 = call-poly <userlib>:"Strip Path Extension__ogtk.vi"("path"=w442) -> ("extension"=w445:string)  [unwired: 1 out]
                n183 = Equal?(x="exe", y=w445) -> (x = y?=w443:bool)
                n184 = case shown="False" w443 {
                  tunnel: w442 -> [w456 w458]
                  tunnel: [w456 w457] -> w441
                  frame False {
                  }
                  frame True {
                    n185 = Strip Path(path=w458) -> (stripped path=w457:path)  [unwired: 1 out]
                  }
                }
                n186 = Array To Spreadsheet String(array=w451, 3:"%s" ("format string")) -> (spreadsheet string=w447:string)  [unwired: 1 in]
                n187 = Build Path(base path=w441, name or relative path="delay_ring.txt") -> (appended path=w452:path)
                n188 = call <vilib>:"Trim Whitespace.vi"("string"=w447) -> ("trimmed string"=w446:string)  [unwired: 1 in]
                n189 = Write to Text File(file (use dialog)=w452, text=w446) -> ()  [unwired: 2 in, 3 out]
              }
            }
          }
          frame #1 {
            n190 = property on="Add Delay" class="Bool (strict)"("Value"=FALSE ("Add Delay")) -> ()  [unwired: 2 in, 2 out]
          }
        }
      }
    }
    n191 = Index Array(array=w155, index (row)=w267, index (col)=w267) -> (element=w266:variant)
    n192 = Or(x=w218, y=w220) -> (x .or. y?=w219:bool)
    n193 = xnode "Read/Write Control"("FPGA VI Reference In"=w237, "error in"=w236, "One Shot"="One Shot Mode", "Reset One Shot"="Rearm Trigger") -> ("FPGA VI Reference Out"=w230:refnum<k20>, "error out"=w229:errorcluster)
    n194 = xnode "Database Variant To Data"("database variant"=w276, "type"=w269) -> ("data"=w196:dbl)  [unwired: 1 in, 1 out]
    n195 = xnode "Database Variant To Data"("database variant"=w277, "type"=w269) -> ("data"=w197:dbl)  [unwired: 1 in, 1 out]
    n196 = xnode "Database Variant To Data"("database variant"=w274, "type"=w269) -> ("data"=w195:dbl)  [unwired: 1 in, 1 out]
    n197 = xnode "Database Variant To Data"("database variant"=w275, "type"=w269) -> ("data"=w194:dbl)  [unwired: 1 in, 1 out]
    n198 = xnode "Database Variant To Data"("database variant"=w272, "type"=w269) -> ("data"=w193:dbl)  [unwired: 1 in, 1 out]
    n199 = xnode "Database Variant To Data"("database variant"=w273, "type"=w269) -> ("data"=w192:dbl)  [unwired: 1 in, 1 out]
    n200 = xnode "Database Variant To Data"("database variant"=w271, "type"=w268) -> ("data"=w260:i8)  [unwired: 1 in, 1 out]
    n201 = xnode "Database Variant To Data"("database variant"=w270, "type"=w268) -> ("data"=w259:i8)  [unwired: 1 in, 1 out]
    n202 = Build Array(w196, w197) -> (w263:dbl[])
    n203 = xnode "Database Variant To Data"("database variant"=w266, "type"=0.0) -> ("data"=w191:dbl)  [unwired: 1 in, 1 out]
    "Peletron (MV)" <- w191
    n204 = Build Array(w195, w194) -> (w262:dbl[])
    n205 = Build Array(w193, w192) -> (w261:dbl[])
    n206 = Equal To 0?(x="Delay Ring") -> (x = 0?=w190:bool)
    n207 = xnode "Read/Write Control"("FPGA VI Reference In"=w230, "error in"=w229) -> ("Not Armed?"=w228:bool, "Del Not Armed?"=w184:bool)  [unwired: 2 out]
    n208 = local read "Delay Value"() -> (w189:dbl)
    n209 = call "calc_variables.vi"("var2"=w259, "Peletron"=w191, "var1"=w260, "Mass"=w261, "Charge"=w262, "Velocity"=w263) -> ("Mass out"=w252:dbl[], "Charge out"=w255:dbl[], "Velocity out"=w258:dbl[])  [unwired: 3 in]
    n210 = property on="Rearm Trigger" class="Bool (strict)"(error in=w229, "Value"=FALSE ("Rearm Trigger")) -> ()  [unwired: 1 in, 2 out]
    n211 = Divide(x="Delay Ring", y=0.93) -> (x/y=w226:dbl)
    n212 = Select(t=w189, s=w190, f=w226) -> (s? t:f=w225:dbl)
    n213 = Not(x=w228) -> (.not. x?=→"Armed":bool)
    n214 = Not(x=w184) -> (.not. x?=→"Del Armed":bool)
    n215 = And(x=w190, y=w185) -> (x .and. y?=w186:bool)
    n216 = property on="Peletron (MV)" class="DigNum (strict)"() -> ("Value"=w264:dbl)  [unwired: 2 in, 2 out]
    n217 = case shown="True" w186 {
      selector: w186 -> [w418 _]
      tunnel: w189 -> [_ w420]
      tunnel: [w418 w419] -> w187
      frame False {
      }
      frame True {
        n218 = call-poly <userlib>:"Data Changed__ogtk.vi"("DBL"=w420) -> ("Changed"=w419:bool)
      }
    }
    n219 = To Fixed-Point(number=w225) -> (fixed-point=w239:fxp<+,16,7>)  [unwired: 1 in]
    n220 = Index Array(array=w255, index #1=0 ("index"), index #2=1 ("index")) -> (element #1=w247:dbl, element #2=w246:dbl)
    "High Charge Limit (fC)" <- w246
    "Low Charge Limit (fC)" <- w247
    n221 = Index Array(array=w258, index #1=0 ("index"), index #2=1 ("index")) -> (element #1=w249:dbl, element #2=w248:dbl)
    "High Velocity" <- w248
    "Low Velocity" <- w249
    n222 = Index Array(array=w252, index #1=0 ("index"), index #2=1 ("index")) -> (element #1=w245:dbl, element #2=w244:dbl)
    "Low Mass (kg)" <- w245
    "High Mass (kg)" <- w244
    n223 = Bundle("Numeric"=w249, "Numeric"=w248, "Numeric"=w247, "Numeric"=w246, "Numeric"=w245, "Numeric"=w244, w243, 26666666.66666667, "Value"=w264, w239, w185) -> (w296:T7)  [unwired: 1 in]
    n224 = call "process_limits.vi"("old output cluster"=w303, "Input cluster"=w296) -> ("Update FPGA"=w242:bool, "output cluster"=w304:T8)  [unwired: 8 in]
    n225 = Unbundle By Name(w304) -> ("Low Velocity Count"=w292:i32, "High Velocity Count"=w291:i32, "Low Charge Limit (ADC ticks)"=w289:i16, "High Charge Limit (ADC ticks)"=w290:i16, "Low Mass (ADC*cycle^2)"=w294:i64, "High Mass (ADC*cycle^2)"=w295:i64, "Mult"=w238:fxp<+,16,7>)
    "Low velocity count" <- w292
    "High velocity count" <- w291
    "High Charge Limit" <- w290
    "Low Charge Limit" <- w289
    "High Mass Limit" <- w295
    "Low Mass Limit" <- w294
    n226 = Or(x=w242, y=w219) -> (x .or. y?=w224:bool)
    n227 = Or(x="Raise Threshold", y="Lower Threshold") -> (x .or. y?=w198:bool)
    n228 = Or(x=w198, y=w224) -> (x .or. y?=w199:bool)
    n229 = Build Array("Filter1 Threshold", "Filter2 Threshold", "Filter3 Threshold", "Filter4 Threshold", "Filter5 Threshold", "Filter6 Threshold", "Filter7 Threshold") -> (w165:i32[])
    n230 = Or(x=w199, y=w187) -> (x .or. y?=w188:bool)
    "Updating FPGA" <- w188
    n231 = Build Array("Threshold 1", "Threshold 2", "Threshold 3", "Threshold 4", "Threshold 5", "Threshold 6", "Threshold 7") -> (w172:bool[])
    n232 = Initialize Array("Update All", 7 ("dimension size")) -> (w173:bool[])
    n233 = Or(x=w173, y=w172) -> (x .or. y?=w166:bool[])
    n234 = Initialize Array("Update By", 7 ("dimension size")) -> (w167:i32[])
    n235 = case shown="True" "Raise Threshold" {
      tunnel: w165 -> [_ w394]
      tunnel: w166 -> [_ w395]
      tunnel: w167 -> [_ w393]
      frame False {
      }
      frame True {
        n236 = Index Array(array=w395) -> (element #1=w416:bool, element #2=w415:bool, element #3=w414:bool, element #4=w413:bool, element #5=w412:bool, element #6=w411:bool, element #7=w410:bool)  [unwired: 7 in]
        n237 = Subtract(x=w394, y=w393) -> (x-y=w417:i32[])
        n238 = Select(t=w417, s=w416, f=w394) -> (s? t:f=w409:i32[])
        n239 = Select(t=w417, s=w415, f=w394) -> (s? t:f=w405:i32[])
        n240 = Select(t=w417, s=w411, f=w394) -> (s? t:f=w398:i32[])
        n241 = Select(t=w417, s=w413, f=w394) -> (s? t:f=w402:i32[])
        n242 = Select(t=w417, s=w412, f=w394) -> (s? t:f=w400:i32[])
        n243 = Select(t=w417, s=w410, f=w394) -> (s? t:f=w396:i32[])
        n244 = Select(t=w417, s=w414, f=w394) -> (s? t:f=w404:i32[])
        n245 = Index Array(array=w405, index=1) -> (element=w390:i32)
        n246 = Index Array(array=w409, index=0) -> (element=w391:i32)
        n247 = Index Array(array=w396, index=6) -> (element=w385:i32)
        n248 = Index Array(array=w400, index=4) -> (element=w387:i32)
        n249 = Index Array(array=w404, index=2) -> (element=w389:i32)
        n250 = Index Array(array=w402, index=3) -> (element=w388:i32)
        n251 = Index Array(array=w398, index=5) -> (element=w386:i32)
        n252 = local write "Filter1 Threshold"(w391) -> ()
        n253 = local write "Filter6 Threshold"(w386) -> ()
        n254 = local write "Filter5 Threshold"(w387) -> ()
        n255 = local write "Filter7 Threshold"(w385) -> ()
        n256 = local write "Filter3 Threshold"(w389) -> ()
        n257 = local write "Filter2 Threshold"(w390) -> ()
        n258 = local write "Filter4 Threshold"(w388) -> ()
        n259 = local write "Raise Threshold"(FALSE ("Raise Threshold")) -> ()
      }
    }
    n260 = case shown="False" "Lower Threshold" {
      tunnel: w165 -> [w350 w374]
      tunnel: w167 -> [_ w384]
      tunnel: w166 -> [_ w383]
      tunnel: [w350 w351] -> w164
      frame False {
      }
      frame True {
        n261 = Index Array(array=w383) -> (element #1=w381:bool, element #2=w380:bool, element #3=w379:bool, element #4=w378:bool, element #5=w377:bool, element #6=w376:bool, element #7=w375:bool)  [unwired: 7 in]
        n262 = Add(x=w374, y=w384) -> (x+y=w382:i32[])
        n263 = Select(t=w382, s=w381, f=w374) -> (s? t:f=w373:i32[])
        n264 = Select(t=w382, s=w380, f=w374) -> (s? t:f=w369:i32[])
        n265 = Select(t=w382, s=w376, f=w374) -> (s? t:f=w362:i32[])
        n266 = Select(t=w382, s=w378, f=w374) -> (s? t:f=w366:i32[])
        n267 = Select(t=w382, s=w377, f=w374) -> (s? t:f=w364:i32[])
        n268 = Select(t=w382, s=w375, f=w374) -> (s? t:f=w360:i32[])
        n269 = Select(t=w382, s=w379, f=w374) -> (s? t:f=w368:i32[])
        n270 = Index Array(array=w369, index=1) -> (element=w357:i32)
        n271 = Index Array(array=w373, index=0) -> (element=w358:i32)
        n272 = Index Array(array=w360, index=6) -> (element=w352:i32)
        n273 = Index Array(array=w364, index=4) -> (element=w354:i32)
        n274 = Index Array(array=w368, index=2) -> (element=w356:i32)
        n275 = Index Array(array=w366, index=3) -> (element=w355:i32)
        n276 = Index Array(array=w362, index=5) -> (element=w353:i32)
        n277 = local write "Filter4 Threshold"(w355) -> ()
        n278 = local write "Filter6 Threshold"(w353) -> ()
        n279 = local write "Filter3 Threshold"(w356) -> ()
        n280 = local write "Filter5 Threshold"(w354) -> ()
        n281 = local write "Filter7 Threshold"(w352) -> ()
        n282 = local write "Filter2 Threshold"(w357) -> ()
        n283 = local write "Filter1 Threshold"(w358) -> ()
        n284 = local write "Lower Threshold"(FALSE ("Lower Threshold")) -> ()
        n285 = Build Array(w358, w357, w356, w355, w354, w353, w352) -> (w351:i32[])
      }
    }
    n286 = Index Array(array=w164) -> (element #1=w212:i32, element #2=w210:i32, element #3=w208:i32, element #4=w206:i32, element #5=w204:i32, element #6=w202:i32, element #7=w200:i32)  [unwired: 7 in]
    n287 = case shown="True" w188 {
      tunnel: w237 -> [w467 w495]
      tunnel: w236 -> [w468 w494]
      tunnel: [w467 w493] -> w321
      tunnel: [w468 w492] -> w320
      tunnel: w212 -> [_ w474]
      tunnel: w210 -> [_ w475]
      tunnel: w208 -> [_ w473]
      tunnel: w206 -> [_ w472]
      tunnel: w204 -> [_ w471]
      tunnel: w202 -> [_ w470]
      tunnel: w200 -> [_ w469]
      tunnel: [w466 w478] -> w301
      tunnel: w295 -> [_ w484]
      tunnel: w294 -> [_ w483]
      tunnel: w292 -> [_ w482]
      tunnel: w291 -> [_ w481]
      tunnel: w290 -> [_ w480]
      tunnel: w289 -> [_ w479]
      tunnel: w302 -> [w466 _]
      tunnel: w238 -> [_ w476]
      frame False {
      }
      frame True {
        n288 = xnode "Read/Write Control"("FPGA VI Reference In"=w495, "error in"=w494, "Low Velocity Count"=w482, "High Velocity Count"=w481, "Filter 1 threshold"=w474, "Filter 2 threshold"=w475, "Filter 3 threshold"=w473, "Filter 4 threshold"=w472, "Filter 5 threshold"=w471, "Filter 6 threshold"=w470, "Filter 7 threshold"=w469, "High Charge Limit"=w480, "Low Charge Limit"=w479, "High Mass Limit"=w484, "Low Mass Limit"=w483, "Mult1"=w476) -> ("FPGA VI Reference Out"=w493:refnum<k20>, "error out"=w492:errorcluster, "Filter 1 Detector 3 Correlation"=w491:i32, "Filter 2 Detector 3 Correlation"=w490:i32, "Filter 3 Detector 3 Correlation"=w489:i32, "Filter 4 Detector 3 Correlation"=w488:i32, "Filter 5 Detector 3 Correlation"=w487:i32, "Filter 6 Detector 3 Correlation"=w486:i32, "Filter 7 Detector 3 Correlation"=w485:i32)
        n289 = Get Date/Time In Seconds() -> (seconds since 1Jan1904=→"Last Update:":timestamp)
        n290 = Bundle("Filter 1 Detector 3 Correlation"=w491, "Filter 2 Detector 3 Correlation"=w490, "Filter 3 Detector 3 Correlation"=w489, "Filter 4 Detector 3 Correlation"=w488, "Filter 5 Detector 3 Correlation"=w487, "Filter 6 Detector 3 Correlation"=w486, "Filter 7 Detector 3 Correlation"=w485) -> (w478:T9)  [unwired: 1 in]
      }
    }
    n291 = call "filter_peaks.vi"("Correlation cluster"=w301, "Filter peak cluster"=w297, "Zero out"="Zero Peak Values", "Run Mode"="Run Mode") -> ("Blinking"=w288:bool, "status"=w293:T2, "Filter peak output"=w298:T5)  [unwired: 5 in]
    n292 = shared-variable "My Computer\\Network Shared Variables.lvlib\\FPGA Trigger"() -> ()  [unwired: 1 in, 2 out]
    n293 = Unbundle By Name(w298) -> ("Filter 1 Peak"=w318:i32, "Filter 2 Peak"=w317:i32, "Filter 3 Peak"=w316:i32, "Filter 4 Peak"=w315:i32, "Filter 5 Peak"=w314:i32, "Filter 6 Peak"=w313:i32, "Filter 7 Peak"=w312:i32)
    "Filter 1 Peak" <- w318
    "Filter 2 Peak" <- w317
    "Filter 3 Peak" <- w316
    "Filter 4 Peak" <- w315
    "Filter 5 Peak" <- w314
    "Filter 6 Peak" <- w313
    "Filter 7 Peak" <- w312
    n294 = property on="Filter 3 Peak" class="DigNum (strict)"("DisabledEnum"=w293, "Blinking"=w288) -> ()  [unwired: 2 in, 2 out]
    n295 = property on="Filter 4 Peak" class="DigNum (strict)"("DisabledEnum"=w293, "Blinking"=w288) -> ()  [unwired: 2 in, 2 out]
    n296 = property on="Filter 7 Peak" class="DigNum (strict)"("DisabledEnum"=w293, "Blinking"=w288) -> ()  [unwired: 2 in, 2 out]
    n297 = property on="Filter 5 Peak" class="DigNum (strict)"("DisabledEnum"=w293, "Blinking"=w288) -> ()  [unwired: 2 in, 2 out]
    n298 = property on="Filter 6 Peak" class="DigNum (strict)"("DisabledEnum"=w293, "Blinking"=w288) -> ()  [unwired: 2 in, 2 out]
    n299 = property on="Filter 2 Peak" class="DigNum (strict)"("DisabledEnum"=w293, "Blinking"=w288) -> ()  [unwired: 2 in, 2 out]
    n300 = property on="Filter 1 Peak" class="DigNum (strict)"("DisabledEnum"=w293, "Blinking"=w288) -> ()  [unwired: 2 in, 2 out]
    n301 = local read "Update Threshold"() -> (w215:bool)
    n302 = call-poly <userlib>:"Data Changed__ogtk.vi"("Boolean"=w215) -> ("Changed"=w216:bool)
    n303 = And(x=w216, y=w215) -> (x .and. y?=w214:bool)
    n304 = case shown="True" w214 {
      frame False {
      }
      frame True {
        n305 = local write "Update Threshold"(FALSE ("Update Threshold")) -> ()
      }
    }
    n306 = Or(x=w218, y=w215) -> (x .or. y?=w217:bool)
    "Sensitivity" <- w243
  }
  n307 = while {
    stop <- w785 stop-if-true
    n308 = case shown="False" "Rate Limiting" {
      frame False {
        n309 = property on="Rearm Trigger" class="Bool (strict)"("DisabledEnum"=T2."Enabled" ("Disabled")) -> ()  [unwired: 2 in, 2 out]
        n310 = property on="One Shot Mode" class="Bool (strict)"("DisabledEnum"=T2."Enabled" ("Disabled")) -> ()  [unwired: 2 in, 2 out]
      }
      frame True {
        n311 = local read "Armed"() -> (w789:bool)
        n312 = Get Date/Time In Seconds() -> (seconds since 1Jan1904=w788:timestamp)
        n313 = property on="Rearm Trigger" class="Bool (strict)"("DisabledEnum"=T2."Disabled and Grayed Out" ("Disabled")) -> ()  [unwired: 2 in, 2 out]
        n314 = case shown="False" w789 {
          tunnel: [w796 FALSE] -> w793
          tunnel: w788 -> [w795 _]
          frame False {
            n315 = flat-sequence {
              tunnel: w795 -> [w797]
              tunnel: [w797] -> w794
              tunnel: [TRUE] -> w796
              tunnel: w794 -> [w803]
              frame #0 {
                n316 = Multiply(x="Min. Time\nBetween Shots (s)", y=1000.0) -> (x*y=w800:dbl)
                n317 = Round Toward +Infinity(x=w800) -> (ceil(x): smallest int >= x=w798:dbl)
                n318 = Wait (ms)(milliseconds to wait=w798) -> ()  [unwired: 1 out]
              }
              frame #1 {
                n319 = Get Date/Time In Seconds() -> (seconds since 1Jan1904=w804:timestamp)
                n320 = Subtract(x=w804, y=w803) -> (x-y=→"Time Betwee Shots":dbl)
              }
            }
          }
          frame True {
          }
        }
        n321 = property on="One Shot Mode" class="Bool (strict)"("DisabledEnum"=T2."Disabled and Grayed Out" ("Disabled"), "Value"=TRUE ("One Shot Mode")) -> ()  [unwired: 2 in, 2 out]
        n322 = local write "Rearm Trigger"(w793) -> ()
      }
    }
    n323 = property on="stopping" class="Bool (strict)"() -> ("Value"=w785:bool)  [unwired: 2 in, 2 out]
  }
  n324 = call "connect out.vi"("error in (no error)"=w41, "connection reference"=w43) -> ()  [unwired: 9 in, 1 out]
  n325 = xnode "Close FPGA VI Reference"("FPGA VI Reference In"=w66, "error in"=w65) -> ("error out"=w68:errorcluster)
  n326 = call <vilib>:"General Error Handler.vi"("error in (no error)"=w68) -> ()  [unwired: 10 in, 5 out]
